vi "LVClass_HasoSlopes Get aliasing.vi"(0 "HasoSlopes in":refnum<class "HasoSlopes.lvclass">, 5 "radius_of_curvature_mm":sgl, 11 "error in (no error)":errorcluster) -> (4 "HasoSlopes out":refnum<class "HasoSlopes.lvclass">, 6 "aliasing":bool, 15 "error out":errorcluster)   [LabVIEW 2020, in "HasoSlopes.lvclass"]
doc: "Test whether slopes will cause aliasing.\n\n--------------------------------------------------------------------------------\n\n<B>HasoSlopesIn </B> : HasoSlopes object.\n<B>HasoSlopesOut </B> : HasoSlopes object.\n<B>radius_of_curvature </B> : radius of curvature of the slopes (mm).\n<B>aliasing </B> : has aliasing (value 0 or 1).\n<B>ErrorIn </B> : Error\n<B>ErrorOut </B> : Error\n\n--------------------------------------------------------------------------------"
uses:
  HasoSlopes.lvclass
  HasoSlopes.lvclass/HasoSlopes.ctl
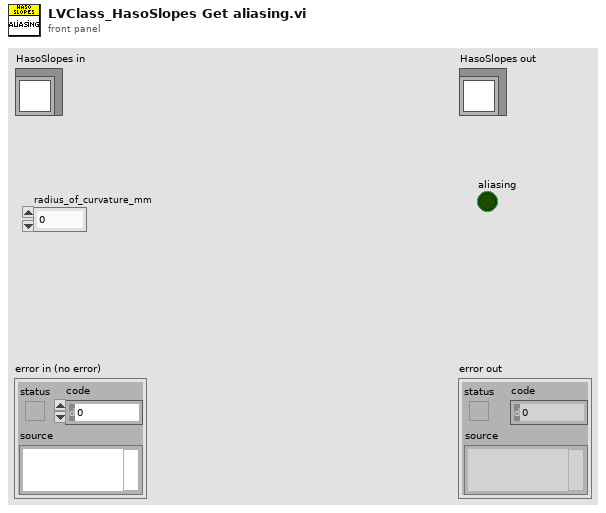
[diagram p1: front panel]
types:
  T1 = typedef "ClassID.ctl" = i64
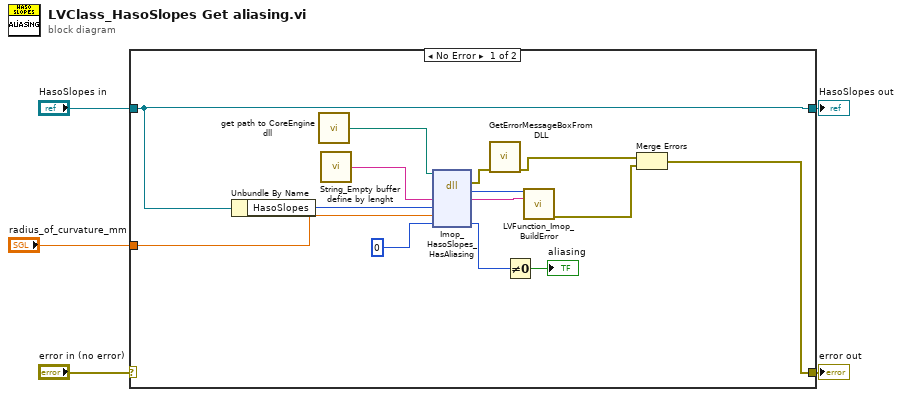
[diagram p0: block diagram]
diagram:
  n1 = case shown="No Error" "error in (no error)" {
    selector: "error in (no error)" -> [_ w21]
    tunnel: [w11 w20] -> w3
    tunnel: "HasoSlopes in" -> [w11 w20]
    tunnel: [w10 w21] -> w2
    tunnel: "radius_of_curvature_mm" -> [w6 _]
    frame No Error {
      n2 = Unbundle By Name(w11) -> ("HasoSlopes"=w17:T1)
      n3 = call "get path to CoreEngine dll.vi"() -> ("path to wavekit library"=w16:path)  [unwired: 14 in, 1 out]
      n4 = call "String_Empty buffer define by lenght.vi"() -> ("Empty buffer"=w14:string)  [unwired: 1 in]
      n5 = dll-call lib="D:/2_trunk/Soft_haso/ImOpCoreEngine4_LV2011/DLLs/ImopEngine4_vc100.dll" fn="Imop_HasoSlopes_HasAliasing"(path in=w16, "message"=w14, "objet"=w17, "radius_of_curvature_mm"=w6, "aliasing"=u8 0) -> (error out=w15:errorcluster, "return type"=w18:i32, "message"=w19:string, "aliasing"=w8:u8)  [unwired: 4 in, 1 out]
      n6 = call "GetErrorMessageBoxFromDLL.vi"("error IN"=w15) -> ("error OUT"=w13:errorcluster)  [unwired: 10 in]
      n7 = Not Equal To 0?(x=w8) -> (x != 0?=→"aliasing":bool)
      n8 = call "LVFunction_Imop_BuildError.vi"("code"=w18, "String to Prepend to source (\"\")"=w19) -> ("error out"=w12:errorcluster)  [unwired: 13 in]
      n9 = Merge Errors(w13, w12) -> (w10:errorcluster)
    }
    frame Error {
    }
  }
  "error out" <- w2
  "HasoSlopes out" <- w3
